vi "handleRejectedCommand.vi"(8 "error in (no error)":errorcluster, 10 "CommandValue":T1, 11 "IModel in":refnum<class "IModel.lvclass">) -> (0 "error out":errorcluster, 3 "IModel out":refnum<class "IModel.lvclass">)   [LabVIEW 2016, in "IModel.lvclass"]
uses:
  IModel.lvclass
  Typedefs/CommandValue.ctl
  Typedefs/SEDSpectrometerTypedefs.lvlib
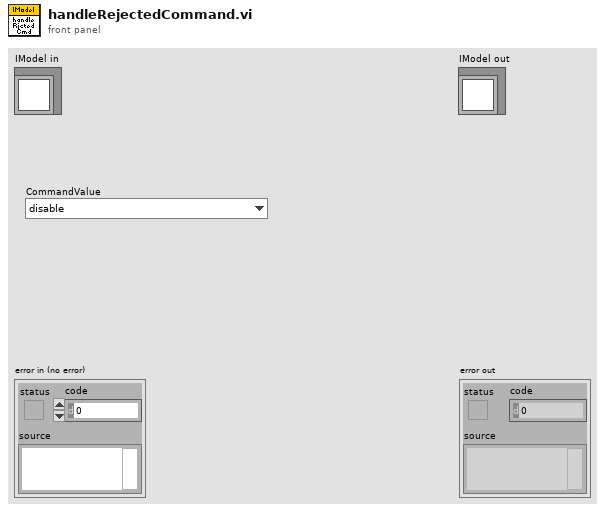
[diagram p1: front panel]
types:
  T1 = typedef "SEDSpectrometerTypedefs.lvlib/CommandValue.ctl" = enum16{"disable", "enable", "exit", "GoToStandby", "OnHeartbeat", "OnIncomingMessagingError", "OnInterrupt", "start", "captureSpectImage", "setSpectTempSetpoint", "stopImageCapture"}
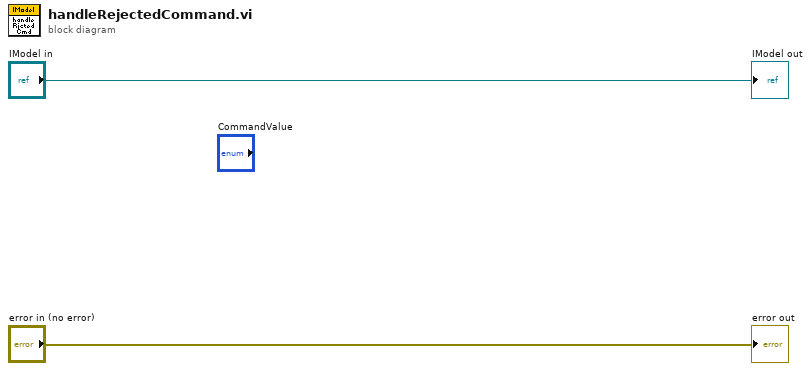
[diagram p0: block diagram]
diagram:
  "error out" <- "error in (no error)"
  "IModel out" <- "IModel in"
